vi "dfd_DFXPSimu AccSub (vector).vi"(5 "quantize output? (T)":bool=TRUE, 7 "op params":T2={"source"=0, "is floating?"=FALSE, "o-mode"=enum."Wrap", "q-mode"=enum."Truncation", "wl"=1, "high limit"=0, "low limit"=0, "iwl"=0, "sign?"=TRUE} {"source" items=["Coef a/k"=0, "Coef b/v"=7, "Input"=1, "Output"=2, "Multiplicand"=3, "Product"=4, "Sum"=5, "Delay"=6, "Gain"=8]}, 8 "filtering statistics in":T6(array[cluster]) {"statistics information"."min value" format="%.2f"; "statistics information"."max value" format="%.2f"; "Quantizer Source" items=["Coefficients a/k"=0, "Coefficients b/v"=7, "Input"=1, "Output"=2, "Multiplicand"=3, "Product"=4, "Sum"=5, "Delay"=6]}, 10 "addends":T7, 11 "acc in":T1={"value"=0, "wl"=0, "iwl"=0, "Signed"=TRUE} {"value" format="%.0x"}) -> (0 "filtering statistics out":T6(array[cluster]) {"statistics information"."min value" format="%.2f"; "statistics information"."max value" format="%.2f"; "Quantizer Source" items=["Coefficients a/k"=0, "Coefficients b/v"=7, "Input"=1, "Output"=2, "Multiplicand"=3, "Product"=4, "Sum"=5, "Delay"=6]}, 3 "acc out":T1={"value"=0, "wl"=0, "iwl"=0, "Signed"=TRUE} {"value" format="%.0x"})   [LabVIEW 2017, in "NI_DigFilter_FXP.lvlib"]
uses:
  <vilib>/addons/Digital Filter Design/NI_DigFilter_FXP.lvlib
  <vilib>/addons/Digital Filter Design/_Objects.llb/dfd_DFXP Data Type (scaler).ctl
  <vilib>/addons/Digital Filter Design/_Objects.llb/dfd_DFXP Data Type (vector).ctl
  <vilib>/addons/Digital Filter Design/_Objects.llb/DFD Quantization Sources.ctl
  <vilib>/addons/Digital Filter Design/_Objects.llb/DFD FXP Statistics Data.ctl
  <vilib>/addons/Digital Filter Design/_Objects.llb/dfd_DFXP Operation Parameter.ctl
  <vilib>/addons/Digital Filter Design/_Objects.llb/dfd_Internal Quantization Srcs.ctl
  <vilib>/addons/Digital Filter Design/NI_DigFilterLicensed.lvlib
panel:
  in  "addend type":T1={"value"=0, "wl"=0, "iwl"=0, "Signed"=TRUE} {"value" format="%.0x"}
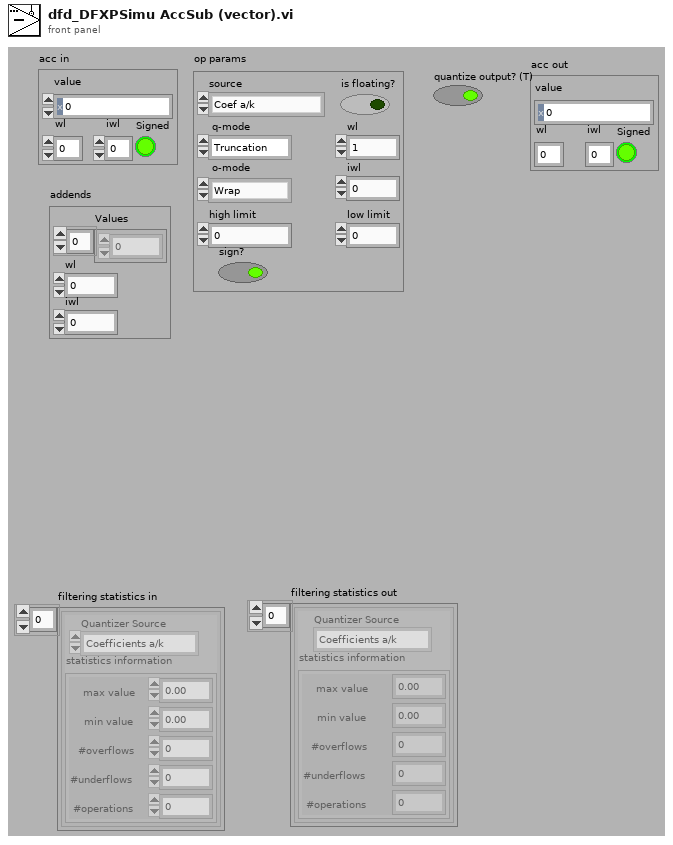
[diagram p1: front panel]
types:
  T1 = typedef "dfd_DFXP Data Type (scaler).ctl" = cluster{"value":i64, "wl":i16, "iwl":i16, "Signed":bool}
  T2 = typedef "dfd_DFXP Operation Parameter.ctl" = cluster{"source":T3, "is floating?":bool, "o-mode":enum16{"Saturation", "Wrap"}, "q-mode":enum16{"Nearest", "Truncation"}, "wl":i16, "high limit":i64, "low limit":i64, "iwl":i16, "sign?":bool}
  T3 = typedef "NI_DigFilterLicensed.lvlib/dfd_Internal Quantization Srcs.ctl" = u16
  T4 = typedef "NI_DigFilterLicensed.lvlib/DFD Quantization Sources.ctl" = u16
  T5 = typedef "NI_DigFilterLicensed.lvlib/DFD FXP Statistics Data.ctl" = cluster{"max value":ext, "min value":ext, "#overflows":i32, "#underflows":i32, "#operations":i32}
  T6 = cluster{"Quantizer Source":T4, "statistics information":T5}[]
  T7 = typedef "dfd_DFXP Data Type (vector).ctl" = cluster{"Values":i64[], "wl":i16, "iwl":i16}
  T8 = cluster{"Quantizer Source":T4, "statistics information":T5}
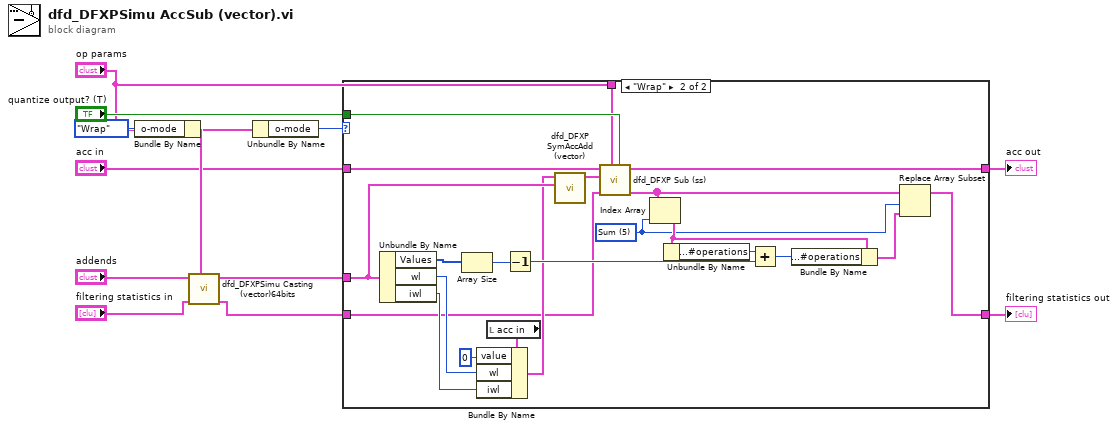
[diagram p0: block diagram]
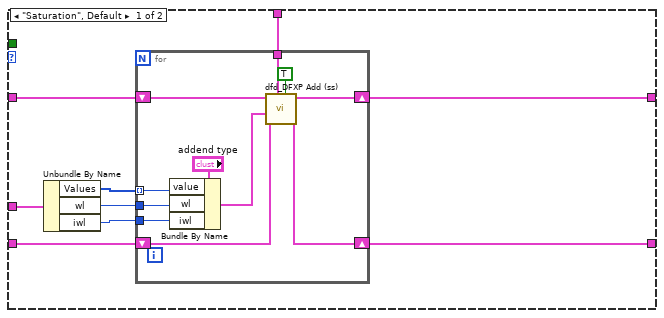
[diagram p2: hidden frame]
diagram:
  n1 = Bundle By Name(cluster="op params", "o-mode"=enum16{"Saturation", "Wrap"}."Wrap" ("o_mode")) -> (w9:T2)
  n2 = call <vilib>:"dfd_DFXPSimu Casting (vector)64bits.vi"("op params"=w9, "filtering statistics in"="filtering statistics in", "Value in"="addends") -> ("filtering statistics out"=w11:T6, "Value out"=w8:T7)  [unwired: 1 in, 6 out]
  n3 = Unbundle By Name("op params") -> ("o-mode"=w10:enum16{"Saturation", "Wrap"})
  n4 = case shown="\"Wrap\"" w10 {
    tunnel: [w21 w34] -> w3
    tunnel: [w20 w46] -> w2
    tunnel: w11 -> [w19 w37]
    tunnel: "acc in" -> [w18 w39]
    tunnel: w8 -> [w17 w54]
    tunnel: "quantize output? (T)" -> [_ w36]
    tunnel: "op params" -> [w13 w35]
    frame "Saturation", Default {
      n5 = Unbundle By Name(w17) -> ("Values"=w16:i64[], "wl"=w15:i16, "iwl"=w14:i16)
      n6 = for {
        tunnel: w13 -> [w29]
        shift-right: [w31] -> w20
        shift-left: w19 -> [w32]
        tunnel: w16 -> [w25] mode=indexing
        shift-right: [w30] -> w21
        shift-left: w18 -> [w28]
        tunnel: w15 -> [w24]
        tunnel: w14 -> [w23]
        n7 = Bundle By Name(cluster="addend type", "value"=w25, "wl"=w24, "iwl"=w23) -> (w22:T1)
        n8 = call <vilib>:"dfd_DFXP Add (ss).vi"("quantize output? (T)"=TRUE ("quantize output?"), "op params"=w29, "filtering statistics in"=w32, "Value in 2"=w22, "Value in"=w28) -> ("filtering statistics out"=w31:T6, "Value out"=w30:T1)  [unwired: 5 out]
      }
    }
    frame "Wrap" {
      w48 = T3 5 items=["Coef a/k"=0, "Coef b/v"=7, "Input"=1, "Output"=2, "Multiplicand"=3, "Product"=4, "Sum"=5, "Delay"=6, "Gain"=8] ("source")
      n9 = Unbundle By Name(w54) -> ("Values"=w45:i64[], "wl"=w43:i16, "iwl"=w42:i16)
      n10 = Array Size(array=w45) -> (size(s)=w53:i32)
      n11 = local read "acc in"() -> (w44:T1)
      n12 = Bundle By Name(cluster=w44, "value"=i64 0, "wl"=w43, "iwl"=w42) -> (w40:T1)
      n13 = Decrement(x=w53) -> (x-1=w47:i32)
      n14 = call <vilib>:"dfd_DFXP SymAccAdd (vector).vi"("Values in"=w54, "Acc"=w40) -> ("Value out"=w38:T1)  [unwired: 9 out]
      n15 = call <vilib>:"dfd_DFXP Sub (ss).vi"("quantize output?(T)"=w36, "op params"=w35, "filtering statistics in"=w37, "Value in 2"=w38, "Value in"=w39) -> ("filtering statistics out"=w33:T6, "Value out"=w34:T1)  [unwired: 5 out]
      n16 = Index Array(array=w33, index=w48) -> (element=w50:T8)
      n17 = Unbundle By Name(w50) -> ("statistics information.#operations"=w52:i32)
      n18 = Add(x=w52, y=w47) -> (x+y=w49:i32)
      n19 = Bundle By Name(cluster=w50, "statistics information.#operations"=w49) -> (w51:T8)
      n20 = Replace Array Subset(array=w33, new element=w51, index=w48) -> (w46:T6)
    }
  }
  "acc out" <- w3
  "filtering statistics out" <- w2
